vi "单个流程写入.vi"(5 "简易流程Id":u16(ring), 6 "是否是简易流程":bool, 7 "添加的路径":path, 8 "error in (no error)":errorcluster caption="错误输入（无错误）", 9 "量程":enum16{"低量程", "高量程"}(ring), 10 "测量模式":enum16{"水样测量", "零点核查", "跨度核查", "标样核查", "加标回收"}(ring), 11 "测量参数":u16(ring) items=["总氮"=2, "总磷"=1, "氨氮"=3, "COD"=22]) -> (0 "error out":errorcluster caption="错误输出", 3 "步数":i32)   [LabVIEW 2016, in "斯坦道总氮.lvlib"]
panel:
  out "数组 2":u16[][](array[numeric]) format="0x%04x"
  out "大小":i32
  out "交织的数组":u16[](array[numeric]) format="0x%04x"
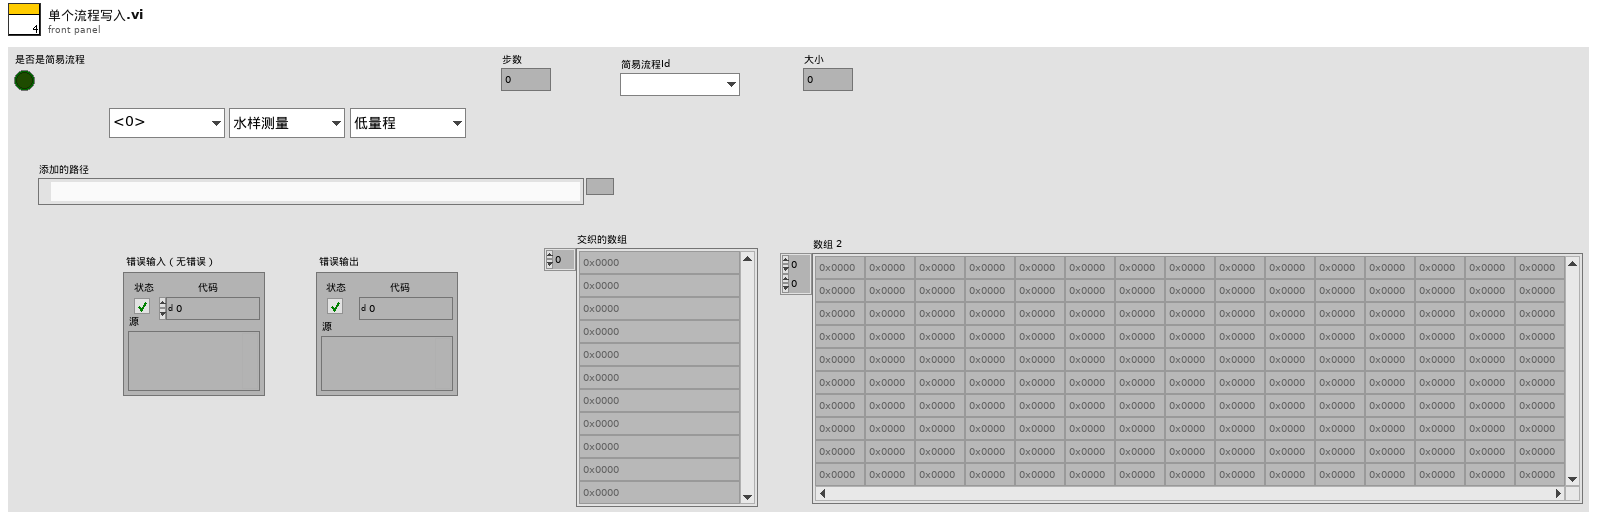
[diagram p1: front panel]
types:
  T1 = cluster{"port":u32, "dac":u8, "adc":u8, "time":u16, "步骤名":string}[]
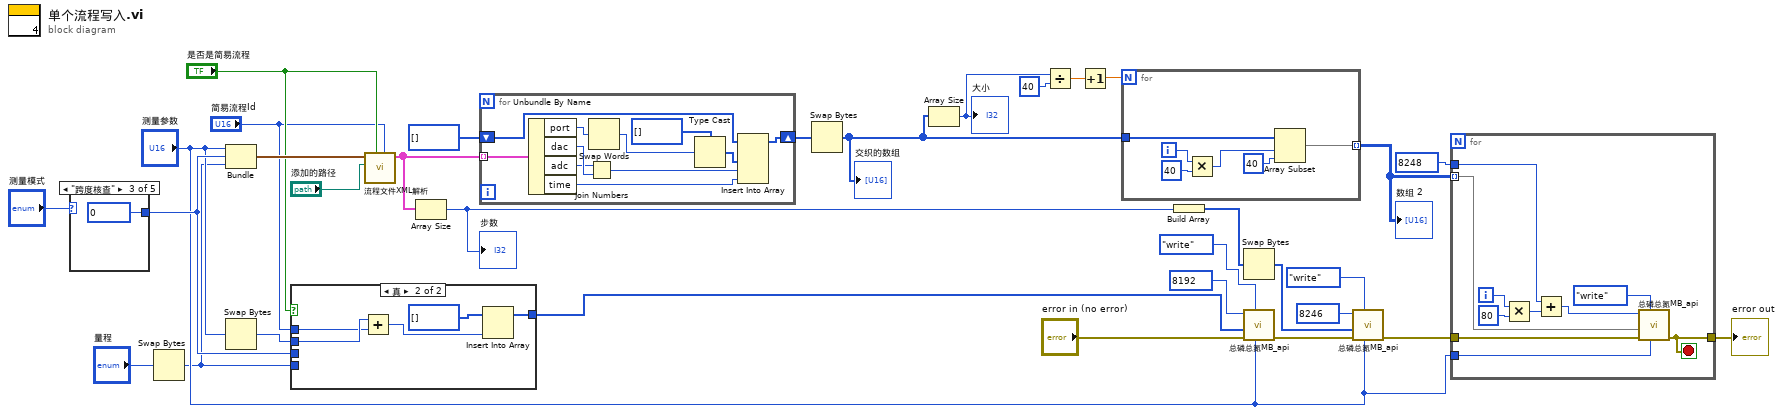
[diagram p0: block diagram]
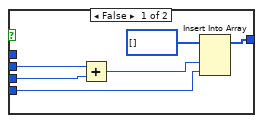
[diagram p2: hidden frame]
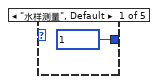
[diagram p3: hidden frame]
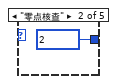
[diagram p4: hidden frame]
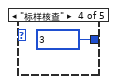
[diagram p5: hidden frame]
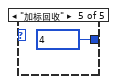
[diagram p6: hidden frame]
diagram:
  n1 = case shown="\"跨度核查\"" "测量模式" {
    tunnel: [u16 1 ("starting address") u16 2 ("starting address") u16 0 ("starting address") u16 3 ("starting address") u16 4 ("starting address")] -> w21
    frame "水样测量", Default {
    }
    frame "零点核查" {
    }
    frame "跨度核查" {
    }
    frame "标样核查" {
    }
    frame "加标回收" {
    }
  }
  n2 = Swap Bytes(anything="量程") -> (byte swapped=w3:u16)
  n3 = Bundle("测量参数"="测量参数", "starting address"=w21, w3) -> (w20:cluster{"测量参数":u16, "starting address":u16, u16})  [unwired: 1 in]
  n4 = Swap Bytes(anything="测量参数") -> (byte swapped=w5:u16)
  n5 = case shown="真" "是否是简易流程" {
    tunnel: [w41 w46] -> w26
    tunnel: w21 -> [w40 _]
    tunnel: w5 -> [w39 w45]
    tunnel: w3 -> [w38 _]
    tunnel: "简易流程Id" -> [_ w44]
    frame False {
      n6 = Add(x=w39, y=w40) -> (x+y=w43:u16)
      n7 = Insert Into Array(array=u16[] [] ("数组"), new element #1=w43, new element #2=w38) -> (w41:u16[])  [unwired: 1 in]
    }
    frame True {
      n8 = Add(x=w45, y=w44) -> (x+y=w48:u16)
      n9 = Insert Into Array(array=u16[] [] ("数组"), new element=w48) -> (w46:u16[])  [unwired: 1 in]
    }
  }
  n10 = call "流程文件XML解析.vi"("简易流程Id"="简易流程Id", "是否是简易流程"="是否是简易流程", "添加的路径"="添加的路径", "参数簇"=w20) -> ("数组"=w12:T1)  [unwired: 7 in]
  n11 = Array Size(array=w12) -> (size(s)=w7:i32)
  "步数" <- w7
  n12 = for {
    tunnel: w12 -> [w59] mode=indexing
    shift-right: [w54] -> w17
    shift-left: u16[] [] -> [w52]
    n13 = Unbundle By Name(w59) -> ("port"=w57:u32, "dac"=w50:u8, "adc"=w49:u8, "time"=w55:u16)
    n14 = Join Numbers(hi=w49, lo=w50) -> ((hi.lo)=w56:u16)
    n15 = Swap Words(1:w57) -> (0:w51:u32)
    n16 = Type Cast(type=u16[] [], x=w51) -> (*(type *) &x=w53:u16[])
    n17 = Insert Into Array(array=w52, new element #1=w53, new element #2=w56, new element #3=w55) -> (w54:u16[])  [unwired: 1 in]
  }
  n18 = Swap Bytes(anything=w17) -> (byte swapped=w14:u16[])
  "交织的数组" <- w14
  n19 = Array Size(array=w14) -> (size(s)=w16:i32)
  "大小" <- w16
  n20 = Divide(x=w16, y=40) -> (x/y=w10:dbl)
  n21 = Increment(x=w10) -> (x+1=w9:dbl)
  n22 = for {
    N: w9 -> [_]
    tunnel: w14 -> [w63]
    tunnel: [w60] -> w13 mode=indexing
    i -> [w65]
    n23 = Multiply(x=w65, y=40) -> (x*y=w62:i32)
    n24 = Array Subset(array=w63, index=w62, length=40 ("y")) -> (w60:u16[])
  }
  "数组 2" <- w13
  n25 = Build Array(w7) -> (w11:i32[])
  n26 = Swap Bytes(anything=w11) -> (byte swapped=w8:i32[])
  n27 = call "总磷总氮MB_api.vi"("Slave ID"="测量参数", "STEP"=enum16{"open", "read", "write", "close"}."write", "Error in"="error in (no error)", "values"=w26, "starting address"=u16 8192) -> ("error out"=w29:errorcluster)  [unwired: 4 in, 2 out]
  n28 = call "总磷总氮MB_api.vi"("Slave ID"="测量参数", "STEP"=enum16{"open", "read", "write", "close"}."write", "Error in"=w29, "values"=w8, "starting address"=u16 8246) -> ("error out"=w25:errorcluster)  [unwired: 4 in, 2 out]
  n29 = for {
    tunnel: u16 8248 ("starting address") -> [w69]
    tunnel: w25 -> [w75]
    tunnel: [w73] -> w23
    tunnel: "测量参数" -> [w72]
    tunnel: w13 -> [w71] mode=indexing
    i -> [w68]
    stop <- w73 stop-if-true
    n30 = Multiply(x=w68, y=80) -> (x*y=w67:i32)
    n31 = Add(x=w69, y=w67) -> (x+y=w70:i32)
    n32 = call "总磷总氮MB_api.vi"("Slave ID"=w72, "STEP"=enum16{"open", "read", "write", "close"}."write", "Error in"=w75, "values"=w71, "starting address"=w70) -> ("error out"=w73:errorcluster)  [unwired: 4 in, 2 out]
  }
  "error out" <- w23
